vi "One Cycle - U8.vi"(1 "In_U8":u8) -> (0 "Out":bool)   [LabVIEW 2015]
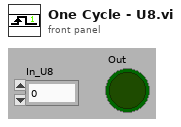
[diagram p1: front panel]
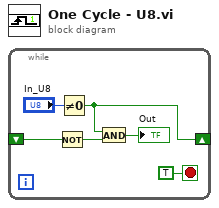
[diagram p0: block diagram]
diagram:
  n1 = while {
    shift-right: [w1] -> _
    shift-left: _ -> [w4]
    stop <- TRUE stop-if-true
    n2 = Not(x=w4) -> (.not. x?=w5:bool)
    n3 = Not Equal To 0?(x="In_U8") -> (x != 0?=w1:bool)
    n4 = And(x=w1, y=w5) -> (x .and. y?=→"Out":bool)
  }
